vi "TestExec.UUT Route Check, Get Inbound Process.vi"(8 "error in (no error)":errorcluster, 10 "parameter name":string="@SN", 11 "UUT SN":string="FB80700274") -> (0 "error out":errorcluster, 1 "No Data":bool, 2 "Connected":bool, 3 "Inbound Process Step":string)   [LabVIEW 2018]
uses:
  <vilib>/addons/database/Auxilliary.llb/DB Tools Parameter Info.ctl
  <vilib>/addons/database/Auxilliary.llb/DB Tools DataTypes.ctl
  <vilib>/addons/database/Auxilliary.llb/DB Tools Parameter Dir.ctl
  <vilib>/addons/database/Connection.llb/DB Tools Open Connec (Path).vi
  <vilib>/addons/database/Connection.llb/Conn Get Properties.vi
  <vilib>/addons/database/Connection.llb/Conn Set Properties.vi
  <vilib>/addons/database/Command.llb/Cmd Execute.vi
  <vilib>/addons/database/Recordset.llb/Rec Fetch Recordset Data (CR).vi
  <vilib>/addons/database/Recordset.llb/Rec Destroy - Command.vi
  <vilib>/addons/database/Command.llb/Cmd Delete.vi
  <vilib>/addons/database/_DB Variant To Data/Database Variant To Data.xnode
  <vilib>/addons/database/NI_Database_API.lvlib
panel:
  out "recordset data":variant[][](array[variant])
  out "Active":bool
  # "FactoryLogix Route Check"
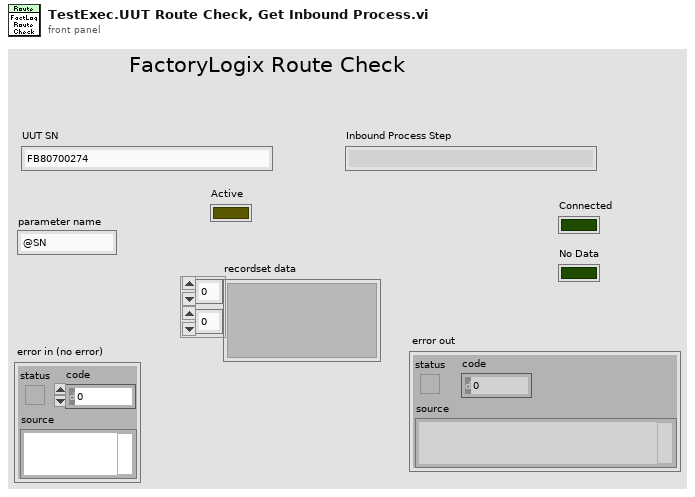
[diagram p1: front panel]
types:
  T1 = enum32{"invalid app kind", "Development System", "Run Time System", "Student Edition", "Embedded LabVIEW", "Evaluation", "Custom"}
  T2 = typedef "NI_Database_API.lvlib/DB Tools DataTypes.ctl" = enum16{"String", "Long (I32)", "Single (SGL)", "Double (DBL)", "Date/Time", "Binary"}
  T3 = typedef "NI_Database_API.lvlib/DB Tools Parameter Dir.ctl" = enum32{"Input", "Output", "Input/Output", "Return Value"}
  T4 = typedef "NI_Database_API.lvlib/DB Tools Parameter Info.ctl" = cluster{"parameter name":string, "type":T2, "direction":T3, "value":variant}
  T5 = typedef "NI_Database_API.lvlib/Conn ObjectReference.ctl" = refnum<k1>
  T6 = typedef "NI_Database_API.lvlib/Conn Properties.ctl" = cluster{"command timeout (s)":i32, "connection string":string, "default database":string, "provider":string}
  T7 = typedef "NI_Database_API.lvlib/Cmd ObjectReference.ctl" = refnum<k1>
  T8 = typedef "NI_Database_API.lvlib/Cmd-Rec Object Reference.ctl" = refnum<k1>
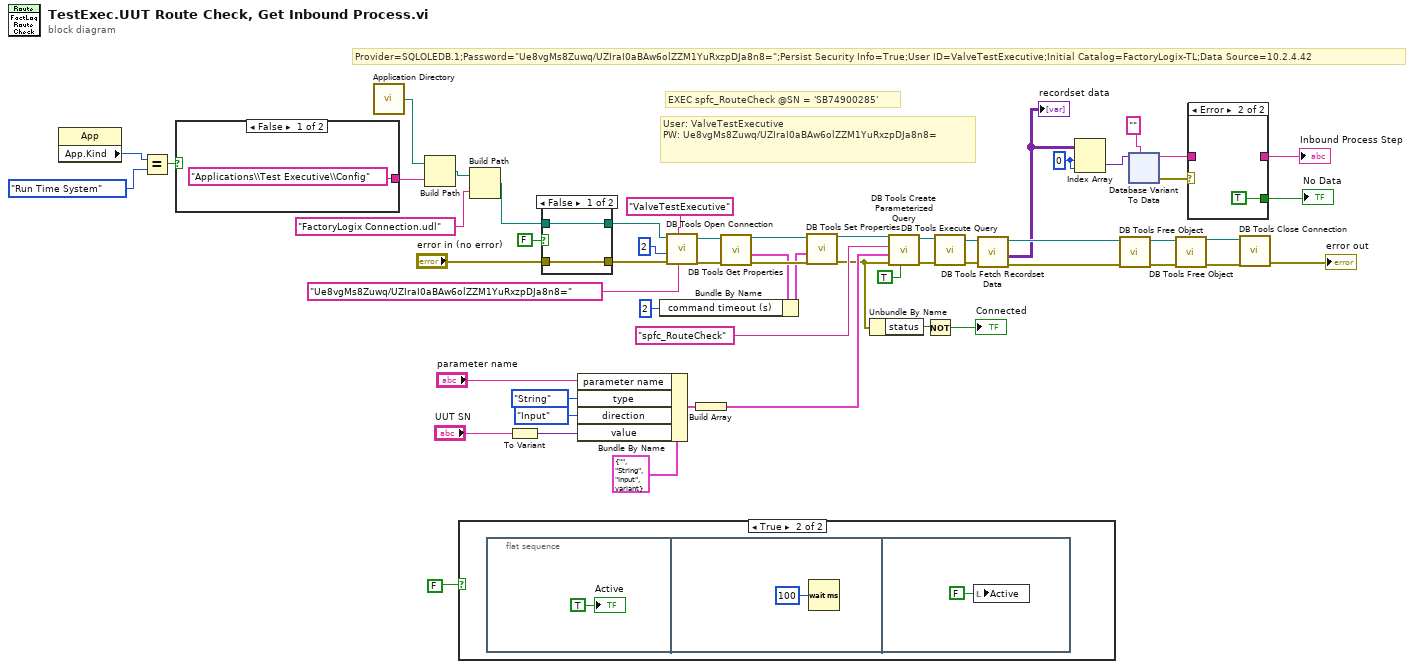
[diagram p0: block diagram]
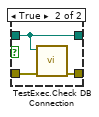
[diagram p2: hidden frame]
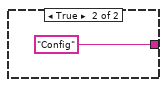
[diagram p3: hidden frame]
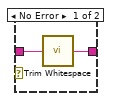
[diagram p4: hidden frame]
diagram:
  w29 = 0 ("index (row)")
  # "Provider=SQLOLEDB.1;Password=\"Ue8vgMs8Zuwq/UZIraI0aBAw6olZZM1YuRxzpDJa8n8=\";Persist Security Info=True;User ID=ValveTestExecutive;Initial Catalog=FactoryLogix-TL;Data Source=10.2.4.42"
  # "EXEC spfc_RouteCheck @SN = 'SB74900285'"
  # "User: ValveTestExecutive\nPW: Ue8vgMs8Zuwq/UZIraI0aBAw6olZZM1YuRxzpDJa8n8="
  n1 = property class="App"() -> ("App.Kind"=w22:T1)  [unwired: 2 in, 2 out]
  n2 = Equal?(x=w22, y=T1."Run Time System" ("Application:Kind")) -> (x = y?=w19:bool)
  n3 = case shown="False" w19 {
    tunnel: ["Applications\\Test Executive\\Config" ("userID") "Config" ("userID")] -> w20
    frame False {
    }
    frame True {
    }
  }
  n4 = call <vilib>:"Application Directory.vi"() -> ("Application Directory"=w38:path)
  n5 = Build Path(base path=w38, name or relative path=w20) -> (appended path=w37:path)
  n6 = case shown="True" FALSE {
    frame False {
    }
    frame True {
      n7 = flat-sequence {
        frame #0 {
          "Active" <- TRUE ("Active")
        }
        frame #1 {
          n8 = Wait (ms)(milliseconds to wait=u32 100) -> ()  [unwired: 1 out]
        }
        frame #2 {
          n9 = local write "Active"(FALSE ("Active")) -> ()
        }
      }
    }
  }
  n10 = Build Path(base path=w37, name or relative path="FactoryLogix Connection.udl" ("userID")) -> (appended path=w5:path)
  n11 = To Variant(anything="UUT SN") -> (Variant=w32:variant)
  n12 = case shown="False" FALSE {
    tunnel: [w63 w66] -> w8
    tunnel: "error in (no error)" -> [w63 w65]
    tunnel: w5 -> [w62 w64]
    tunnel: [w62 w64] -> w4
    frame False {
    }
    frame True {
      n13 = call "TestExec.Check DB Connection.vi"("Error In"=w65, "UDL File (if blank, use Connection String)"=w64) -> ("Error Out"=w66:errorcluster)  [unwired: 8 in, 1 out]
    }
  }
  n14 = Bundle By Name(cluster=T4 {"parameter name"="", "type"=enum."String", "direction"=enum."Input", "value"=variant} ("parameter information"), "parameter name"="parameter name", "type"=DB_Tools_DataTypes."String", "direction"=DB_Tools_Parameter_Dir."Input", "value"=w32) -> (w55:T4)
  n15 = call-poly <vilib>:"DB Tools Open Connection.vi"("password"="Ue8vgMs8Zuwq/UZIraI0aBAw6olZZM1YuRxzpDJa8n8=", "userID"="ValveTestExecutive", "error in (no error)"=w8, "connection timeout (15)"=2, "connection information"=w4) -> ("error out"=w12:errorcluster, "connection reference"=w13:T5)  [unwired: 3 in]
  n16 = Build Array(w55) -> (w56:T4[])
  n17 = call-poly <vilib>:"DB Tools Get Properties.vi"("error in (no error)"=w12, "connection reference"=w13) -> ("error out"=w11:errorcluster, "connection properties"=w10:T6, "connection reference out"=w14:T5)  [unwired: 3 in]
  n18 = Bundle By Name(cluster=w10, "command timeout (s)"=2) -> (w9:T6)
  n19 = call-poly <vilib>:"DB Tools Set Properties.vi"("error in (no error)"=w11, "connection properties"=w9, "connection reference"=w14) -> ("error out"=w17:errorcluster, "connection reference out"=w16:T5)  [unwired: 3 in]
  n20 = Unbundle By Name(w17) -> ("status"=w35:bool)
  n21 = call <vilib>:"DB Tools Create Parameterized Query.vi"("stored procedure? (F)"=TRUE, "error in (no error)"=w17, "parameters"=w56, "SQL query"="spfc_RouteCheck", "connection reference"=w16) -> ("error out"=w48:errorcluster, "command reference"=w49:T7)  [unwired: 2 in, 1 out]
  n22 = Not(x=w35) -> (.not. x?=→"Connected":bool)
  n23 = call-poly <vilib>:"DB Tools Execute Query.vi"("error in (no error)"=w48, "command reference"=w49) -> ("error out"=w46:errorcluster, "command-recordset reference"=w47:T8)  [unwired: 6 in]
  n24 = call-poly <vilib>:"DB Tools Fetch Recordset Data.vi"("error in (no error)"=w46, "command-recordset reference"=w47) -> ("error out"=w40:errorcluster, "recordset data"=w30:variant[][], "command-recordset reference out"=w45:T8)  [unwired: 3 in]
  "recordset data" <- w30
  n25 = Index Array(array=w30, index (row)=w29, index (col)=w29) -> (element=w28:variant)
  n26 = call-poly <vilib>:"DB Tools Free Object.vi"("error in (no error)"=w40, "command-recordset reference"=w45) -> ("error out"=w43:errorcluster, "command reference"=w44:T7)  [unwired: 8 in]
  n27 = xnode "Database Variant To Data"("database variant"=w28, "type"="") -> ("data"=w25:string, "error out"=w26:errorcluster)  [unwired: 1 in]
  n28 = call-poly <vilib>:"DB Tools Free Object.vi"("error in (no error)"=w43, "command reference"=w44) -> ("error out"=w41:errorcluster, "connection reference"=w42:T5)  [unwired: 8 in]
  n29 = case shown="Error" w26 {
    tunnel: w25 -> [w68 _]
    tunnel: [w67 _] -> w24
    tunnel: [_ TRUE] -> w23
    frame No Error {
      n30 = call <vilib>:"Trim Whitespace.vi"("string"=w68) -> ("trimmed string"=w67:string)  [unwired: 1 in]
    }
    frame Error {
    }
  }
  "Inbound Process Step" <- w24
  "No Data" <- w23
  n31 = call <vilib>:"DB Tools Close Connection.vi"("error in (no error)"=w41, "connection reference"=w42) -> ("error out"=→"error out":errorcluster)  [unwired: 5 in]
